vi "COM read file.vi"() -> (2 "COM file path":path, 3 "COM port":refnum<visa-resource-name>)   [LabVIEW 2020]
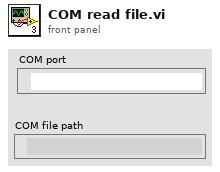
[diagram p1: front panel]
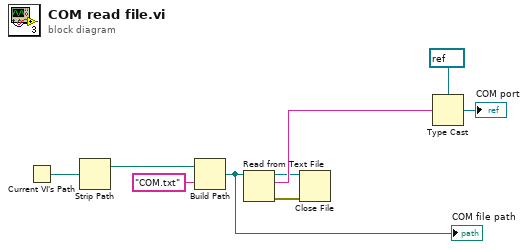
[diagram p0: block diagram]
diagram:
  n1 = Current VI's Path() -> (path=w8:path)
  n2 = Strip Path(path=w8) -> (stripped path=w9:path)  [unwired: 1 out]
  n3 = Build Path(base path=w9, name or relative path="COM.txt") -> (appended path=w6:path)
  "COM file path" <- w6
  n4 = Read from Text File(file (use dialog)=w6) -> (refnum out=w1:refnum<file>, text=w5:string, error out=w2:errorcluster)  [unwired: 3 in, 1 out]
  n5 = Close File(refnum=w1, error in=w2) -> ()  [unwired: 2 out]
  n6 = Type Cast(type=refnum<visa-resource-name> refnum ("COM Port Out"), x=w5) -> (*(type *) &x=→"COM port":refnum<visa-resource-name>)
